vi "Write_GEA3.vi"(0 "session in":refnum<k35>, 5 "board":u8 format="%x", 7 "dst":i64 format="%x", 9 "Write cluster":T2 {"ERD" format="%x"}, 11 "error in (no error)":errorcluster) -> (4 "session out":refnum<k35>, 8 "Write ERD":T1 {"ERD Number" format="%x"}, 15 "error out":errorcluster)   [LabVIEW 2021]
uses:
  Controles/Write_ERD.ctl
  Controles/Read_ERD.ctl
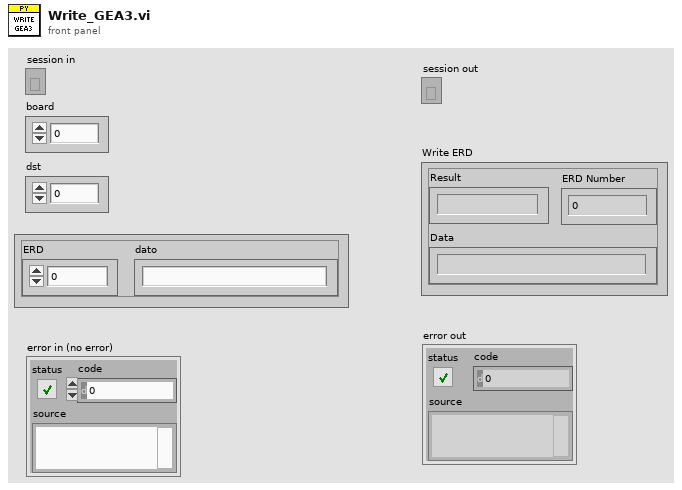
[diagram p1: front panel]
types:
  T1 = typedef "Read_ERD.ctl" = cluster{"Result":string, "ERD Number":i64, "Data":string}
  T2 = typedef "Write_ERD.ctl" = cluster{"ERD":i64, "dato":string}
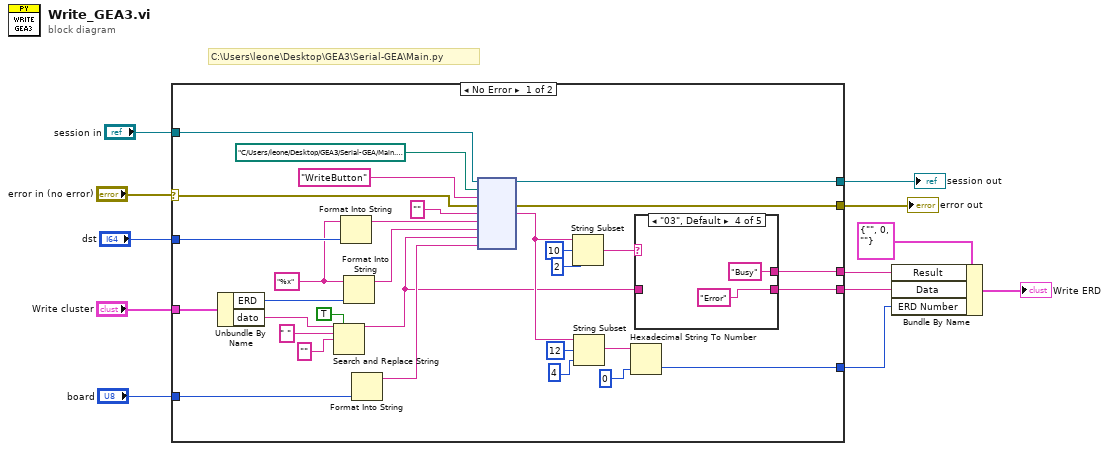
[diagram p0: block diagram]
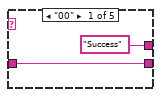
[diagram p2: hidden frame]
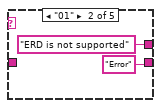
[diagram p3: hidden frame]
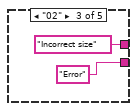
[diagram p4: hidden frame]
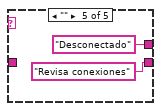
[diagram p5: hidden frame]
diagram:
  # "C:\\Users\\leone\\Desktop\\GEA3\\Serial-GEA\\Main.py"
  n1 = case shown="No Error" "error in (no error)" {
    selector: "error in (no error)" -> [w26 w54]
    tunnel: "dst" -> [w40 _]
    tunnel: "board" -> [w37 _]
    tunnel: "session in" -> [w36 w55]
    tunnel: [w35 w55] -> w9
    tunnel: [w34 w54] -> w8
    tunnel: "Write cluster" -> [w27 _]
    tunnel: [w21 _] -> w4
    tunnel: [w16 _] -> w2
    tunnel: [w14 _] -> w1
    frame No Error {
      w25 = "%x" ("format string")
      n2 = Unbundle By Name(w27) -> ("ERD"=w32:i64, "dato"=w31:string)
      n3 = Search and Replace String(replace all?=TRUE ("replace all? (F)"), input string=w31, search string=" ", replace string="" ("replace string (\"\")")) -> (result string=w13:string)  [unwired: 4 in, 3 out]
      n4 = Format Into String(format string=w25, w40) -> (resulting string=w39:string)  [unwired: 2 in, 1 out]
      n5 = Format Into String(format string=w25, w32) -> (resulting string=w38:string)  [unwired: 2 in, 1 out]
      n6 = Format Into String(w37) -> (resulting string=w33:string)  [unwired: 3 in, 1 out]
      n7 = node(w36, path "C:/Users/leone/Desktop/GEA3/Serial-GEA/Main.py" ("module path"), "WriteButton" ("function name"), w26, "" ("data_hex"), w39, w38, w13, w33) -> (w35:refnum<k35>, w34:errorcluster, w20:string)  [unwired: 4 in, 2 out]
      n8 = String Subset(string=w20, offset (0)=10, length (rest)=2 ("length (rest)")) -> (substring=w22:string)
      n9 = String Subset(string=w20, offset (0)=12, length (rest)=4 ("length (rest)")) -> (substring=w17:string)
      n10 = Hexadecimal String To Number(string=w17, default (0uL)=i64 0) -> (number=w16:i64)  [unwired: 1 in, 1 out]
      n11 = case shown="\"03\", Default" w22 {
        tunnel: ["Success" "ERD is not supported" "Incorrect size" "Busy" "Desconectado"] -> w21
        tunnel: [w44 "Error" ("result string") "Error" ("result string") "Error" ("result string") "Revisa conexiones"] -> w14
        tunnel: w13 -> [w44 _ _ _ _]
        frame "00" {
        }
        frame "01" {
        }
        frame "02" {
        }
        frame "03", Default {
        }
        frame "" {
        }
      }
    }
    frame Error {
    }
  }
  "session out" <- w9
  "error out" <- w8
  n12 = Bundle By Name(cluster=T1 {"Result"="", "ERD Number"=0, "Data"=""} ("Read ERD"), "Result"=w4, "Data"=w1, "ERD Number"=w2) -> (→"Write ERD":T1)
